vi "Format Header.vi"(0 "address":u8 format="%.0x", 5 "write":bool) -> (4 "header":u8 format="%.0x")   [LabVIEW 2013, in "DIO SPI User Library.lvlib"]
doc: "Format read/write command and address into header expected by the slave user logic."
uses:
  DIO SPI User Library.lvlib
panel:
  # "Format read/write command and address into header expected by the slave user logic."
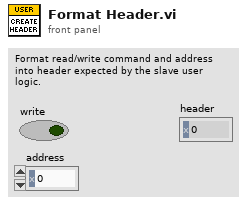
[diagram p1: front panel]
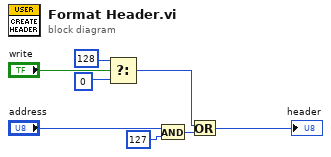
[diagram p0: block diagram]
diagram:
  n1 = Select(t=u8 128 ("Header"), s="write", f=u8 0 ("Header")) -> (s? t:f=w5:u8)
  n2 = And(x="address", y=u8 127 ("Header")) -> (x .and. y?=w1:u8)
  n3 = Or(x=w5, y=w1) -> (x .or. y?=→"header":u8)
